vi "Digital Out.vi"() -> ()   [LabVIEW 2020]
uses:
  <vilib>/DAQmx/write.llb/DAQmx Write (Digital 1D Wfm NChan NSamp).vi
  <vilib>/DAQmx/create/channels.llb/DAQmx Create Channel (DO-Digital Output).vi
  <vilib>/DAQmx/configure/timing.llb/DAQmx Timing (Sample Clock).vi
  <vilib>/Waveform/WDTOps.llb/WDT Append Waveforms DBL.vi
  <vilib>/Waveform/DWDTOps.llb/DWDT Analog to Digital.vi
  <vilib>/Waveform/DWDTOps.llb/DWDT Digital Signal Subset.vi
  <vilib>/Waveform/DWDTOps.llb/DWDT Uncompress Digital.vi
  <vilib>/DAQmx/miscellaneous.llb/DAQmx Fill In Error Info.vi
  <vilib>/measure/NI_MABase.lvlib
  <vilib>/measure/NI_MAPro.lvlib
panel:
  in  "Trigger 2":tag
  in  "Trigger 1":tag
  in  "Trigger-to-\nTrigger Delay (ms)":dbl=200.0 min=0.0 max=1000.0
  out "Digital Waveform Graph":digitalwaveform[](graph)
  in  "Start-to-Block\nDelay (ms)":dbl=1000.0 min=0.0 max=1000.0
  in  "Stim Pulse\nFrequency (Hz)":dbl=1.0 min=0.0
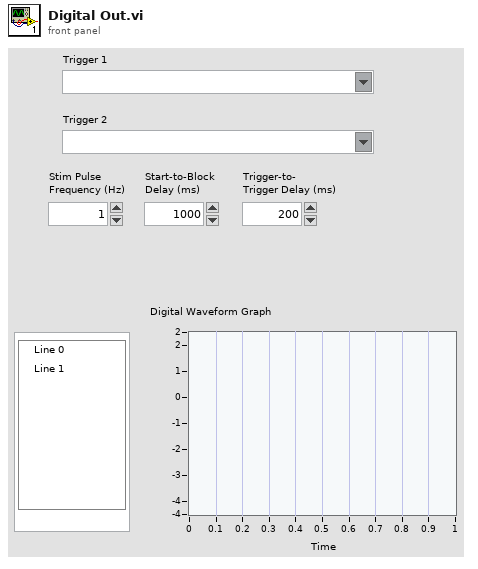
[diagram p1: front panel]
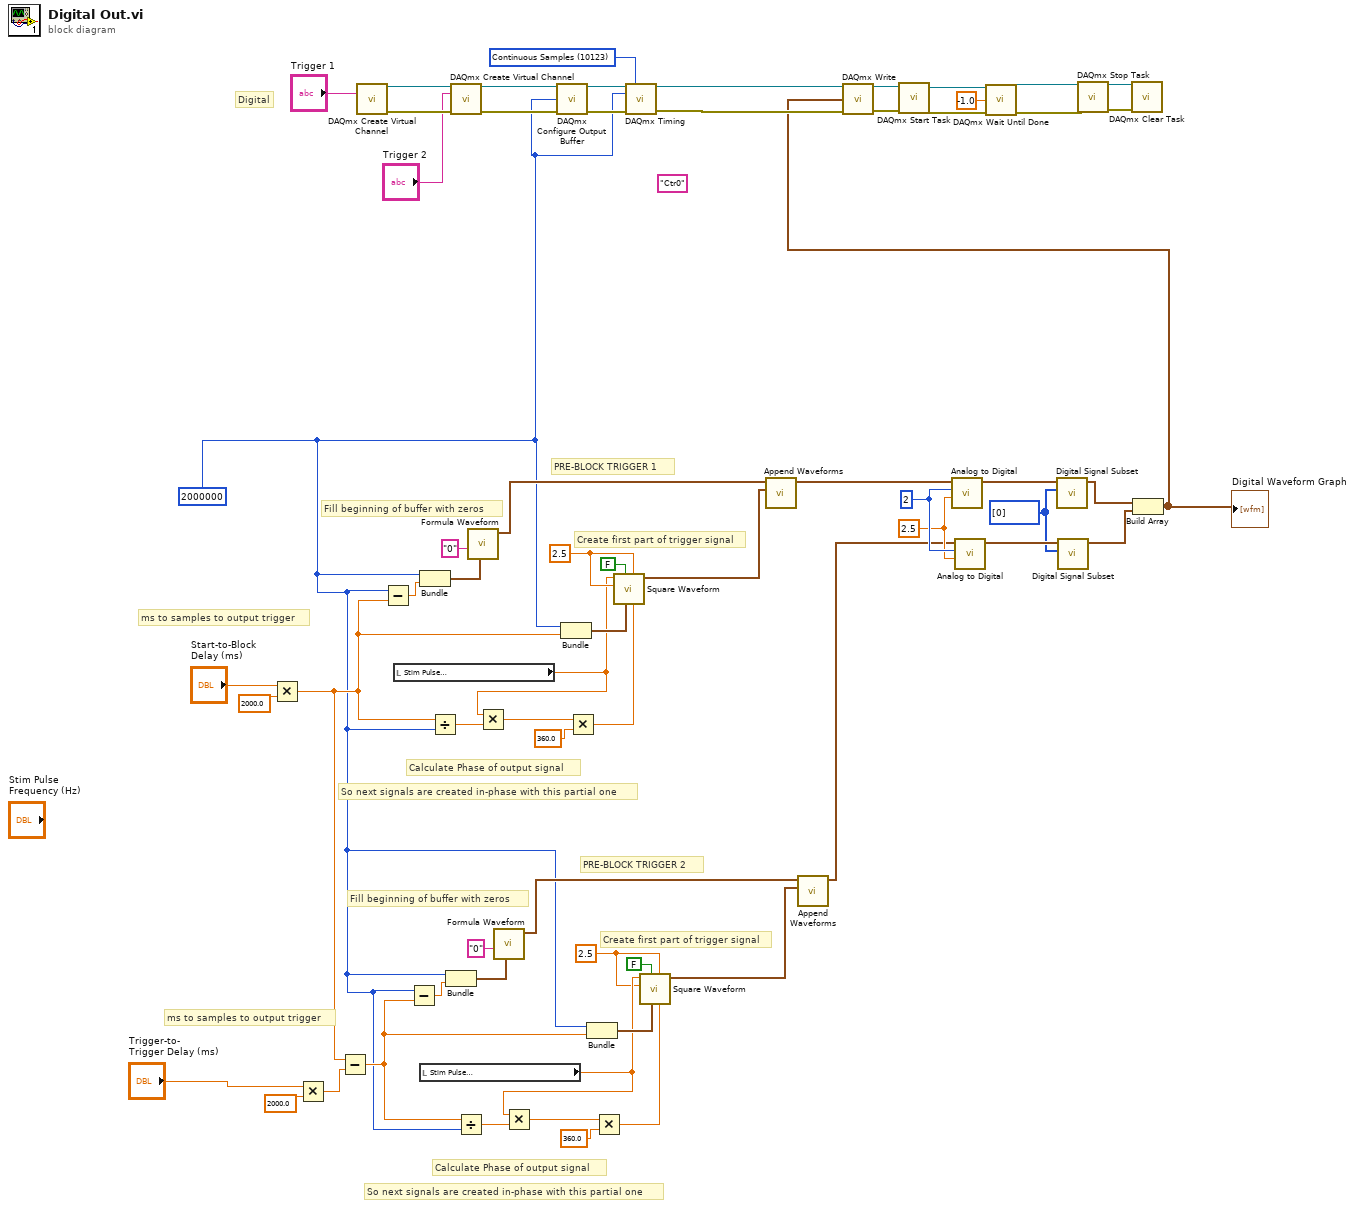
[diagram p0: block diagram]
diagram:
  w8 = 10123 items=["Finite Samples"=10178, "Continuous Samples"=10123, "Hardware Timed Single Point"=12522] ("sample mode")
  (unwired) "Ctr0" ("Local Terminal Name")
  w9 = 2000000 ("x")
  w29 = i32[] [0] ("signals")
  w32 = 2.5 ("full-scale range (pk-pk)")
  w33 = 2 ("resolution (16 bit)")
  w34 = 2.5 ("amplitude")
  w64 = 2.5 ("amplitude")
  # "Digital"
  # "PRE-BLOCK TRIGGER 2"
  # "So next signals are created in-phase with this partial one"
  # "Calculate Phase of output signal"
  # "Create first part of trigger signal"
  # "Fill beginning of buffer with zeros"
  # "ms to samples to output trigger"
  # "PRE-BLOCK TRIGGER 1"
  # "So next signals are created in-phase with this partial one"
  # "Calculate Phase of output signal"
  # "Create first part of trigger signal"
  # "Fill beginning of buffer with zeros"
  # "ms to samples to output trigger"
  n1 = Multiply(x="Start-to-Block\nDelay (ms)", y=2000.0) -> (x*y=w36:dbl)
  n2 = Multiply(x="Trigger-to-\nTrigger Delay (ms)", y=2000.0) -> (x*y=w37:dbl)
  n3 = Subtract(x=w36, y=w37) -> (x-y=w35:dbl)
  n4 = call-poly <vilib>:"DAQmx Create Virtual Channel.vi"("lines"="Trigger 1") -> ("task out"=w20:refnum<k21>, "error out"=w21:errorcluster)  [unwired: 13 in]
  n5 = Subtract(x=w9, y=w36) -> (x-y=w57:dbl)
  n6 = local read "Stim Pulse\nFrequency (Hz)"() -> (w38:dbl)
  n7 = Subtract(x=w9, y=w35) -> (x-y=w46:dbl)
  n8 = Bundle("x"=w9, w57) -> (w59:cluster{"x":i32, dbl})  [unwired: 1 in]
  n9 = local read "Stim Pulse\nFrequency (Hz)"() -> (w40:dbl)
  n10 = Divide(x=w36, y=w9) -> (x/y=w53:dbl)
  n11 = Bundle("x"=w9, w46) -> (w48:cluster{"x":i32, dbl})  [unwired: 1 in]
  n12 = call-poly <vilib>:"DAQmx Create Virtual Channel.vi"("task in"=w20, "lines"="Trigger 2", "error in"=w21) -> ("task out"=w16:refnum<k21>, "error out"=w15:errorcluster)  [unwired: 11 in]
  n13 = Divide(x=w35, y=w9) -> (x/y=w42:dbl)
  n14 = call <vilib>:"Formula Waveform.vi"("sampling info"=w59, "formula"="0") -> ("signal out"=w56:waveform(dbl))  [unwired: 8 in, 1 out]
  n15 = Multiply(x=w38, y=w53) -> (x*y=w52:dbl)
  n16 = call <vilib>:"Formula Waveform.vi"("sampling info"=w48, "formula"="0") -> ("signal out"=w45:waveform(dbl))  [unwired: 8 in, 1 out]
  n17 = Multiply(x=w40, y=w42) -> (x*y=w41:dbl)
  n18 = call <vilib>:"DAQmx Configure Output Buffer.vi"("task/channels in"=w16, "buffer size (in samples per channel)"=w9, "error in"=w15) -> ("task out"=w17:refnum<k21>, "error out"=w18:errorcluster)  [unwired: 11 in]
  n19 = Bundle("x"=w9, w36) -> (w58:cluster{"x":i32, dbl})  [unwired: 1 in]
  n20 = Multiply(x=w52, y=360.0) -> (x*y=w24:dbl)
  n21 = Bundle("x"=w9, w35) -> (w47:cluster{"x":i32, dbl})  [unwired: 1 in]
  n22 = Multiply(x=w41, y=360.0) -> (x*y=w39:dbl)
  n23 = call <vilib>:"Square Waveform.vi"("duty cycle (%)"=w24, "offset"=w64, "sampling info"=w58, "reset signal"=FALSE, "amplitude"=w64, "frequency"=w38) -> ("signal out"=w55:waveform(dbl))  [unwired: 4 in, 1 out]
  n24 = call-poly <vilib>:"DAQmx Timing.vi"("task/channels in"=w17, "sample mode"=w8, "rate"=w9, "error in"=w18) -> ("task out"=w11:refnum<k21>, "error out"=w12:errorcluster)  [unwired: 10 in]
  n25 = call <vilib>:"Square Waveform.vi"("duty cycle (%)"=w39, "offset"=w34, "sampling info"=w47, "reset signal"=FALSE, "amplitude"=w34, "frequency"=w40) -> ("signal out"=w44:waveform(dbl))  [unwired: 4 in, 1 out]
  n26 = call-poly <vilib>:"Append Waveforms.vi"("waveform B"=w55, "waveform A"=w56) -> ("waveform out"=w26:waveform(dbl))  [unwired: 8 in, 1 out]
  n27 = call-poly <vilib>:"Append Waveforms.vi"("waveform B"=w44, "waveform A"=w45) -> ("waveform out"=w25:waveform(dbl))  [unwired: 8 in, 1 out]
  n28 = call-poly <vilib>:"Analog to Digital.vi"("full-scale range (pk-pk)"=w32, "resolution (16 bit)"=w33, "analog waveform"=w26) -> ("digital waveform"=w31:digitalwaveform)  [unwired: 5 in, 3 out]
  n29 = call-poly <vilib>:"Analog to Digital.vi"("full-scale range (pk-pk)"=w32, "resolution (16 bit)"=w33, "analog waveform"=w25) -> ("digital waveform"=w30:digitalwaveform)  [unwired: 5 in, 3 out]
  n30 = call-poly <vilib>:"Digital Signal Subset.vi"("signals"=w29, "digital waveform"=w31) -> ("digital subset"=w28:digitalwaveform)  [unwired: 8 in, 1 out]
  n31 = call-poly <vilib>:"Digital Signal Subset.vi"("signals"=w29, "digital waveform"=w30) -> ("digital subset"=w27:digitalwaveform)  [unwired: 8 in, 1 out]
  n32 = Build Array(w28, w27) -> (w10:digitalwaveform[])
  "Digital Waveform Graph" <- w10
  n33 = call-poly <vilib>:"DAQmx Write.vi"("task/channels in"=w11, "data"=w10, "error in"=w12) -> ("task out"=w14:refnum<k21>, "error out"=w13:errorcluster)  [unwired: 10 in, 1 out]
  n34 = call <vilib>:"DAQmx Start Task.vi"("task/channels in"=w14, "error in"=w13) -> ("task out"=w6:refnum<k21>, "error out"=w5:errorcluster)  [unwired: 12 in]
  n35 = call <vilib>:"DAQmx Wait Until Done.vi"("task/channels in"=w6, "timeout (sec)"=-1.0, "error in"=w5) -> ("task out"=w3:refnum<k21>, "error out"=w4:errorcluster)  [unwired: 11 in]
  n36 = call <vilib>:"DAQmx Stop Task.vi"("task/channels in"=w3, "error in"=w4) -> ("task out"=w2:refnum<k21>, "error out"=w7:errorcluster)  [unwired: 12 in]
  n37 = call <vilib>:"DAQmx Clear Task.vi"("task in"=w2, "error in"=w7) -> ()  [unwired: 13 in, 1 out]
